vi "GEOM_AbsROI.vi"(10 "readmode":string) -> ()   [LabVIEW 2016]
uses:
  GEOM_VAR_action.ctl
  GEOM_Gbls.vi
  DBSHAND/private/vis/DatabaseHand_Element_Set(string).vi
  DBSHAND/private/vis/DatabaseHand_Element_Set(U32).vi
panel:
  out "ysize out":u32
  out "ystart out":u32
  out "xsize out":u32
  out "xstart out":u32
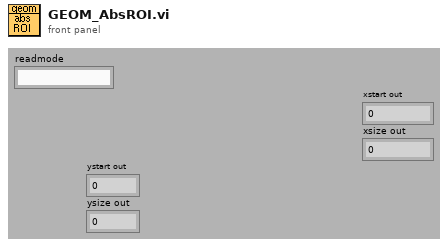
[diagram p1: front panel]
types:
  T1 = typedef "GEOM_FPAReadMode.ctl" = cluster{"name":string, "Amplifiers":T2[]}
  T2 = typedef "GEOM_Amplifier.ctl" = cluster{"number":i32, "type":T3, "rotated":i16, "fliped":u16, "FPAcoord":cluster{"xstart":i32, "ystart":i32}, "Physical_size":cluster{"columns":i32, "rows":i32}, "predata":cluster{"columns":i32, "rows":i32}, "postdata":cluster{"columns":i32, "rows":i32}, "Req ROIs":T4, "Corr ROI":T4, "Detnumber":i32, "ampID":string, "discard":i32}
  T3 = typedef "GEOM_AmpType.ctl" = u16
  T4 = typedef "GEOM_ROI.ctl" = T5[]
  T5 = typedef "GEOM_Coords.ctl" = cluster{"xstart":u32, "ystart":u32, "xsize":u32, "ysize":u32}
  T6 = typedef "GEOM_VAR_action.ctl" = enum16{"read", "write"}
  T7 = cluster{"xstart":i32, "ystart":i32, "xend":i32, "yend":i32}
  T8 = typedef "DatabaseHand_RefNum.ctl" = refnum<vi>
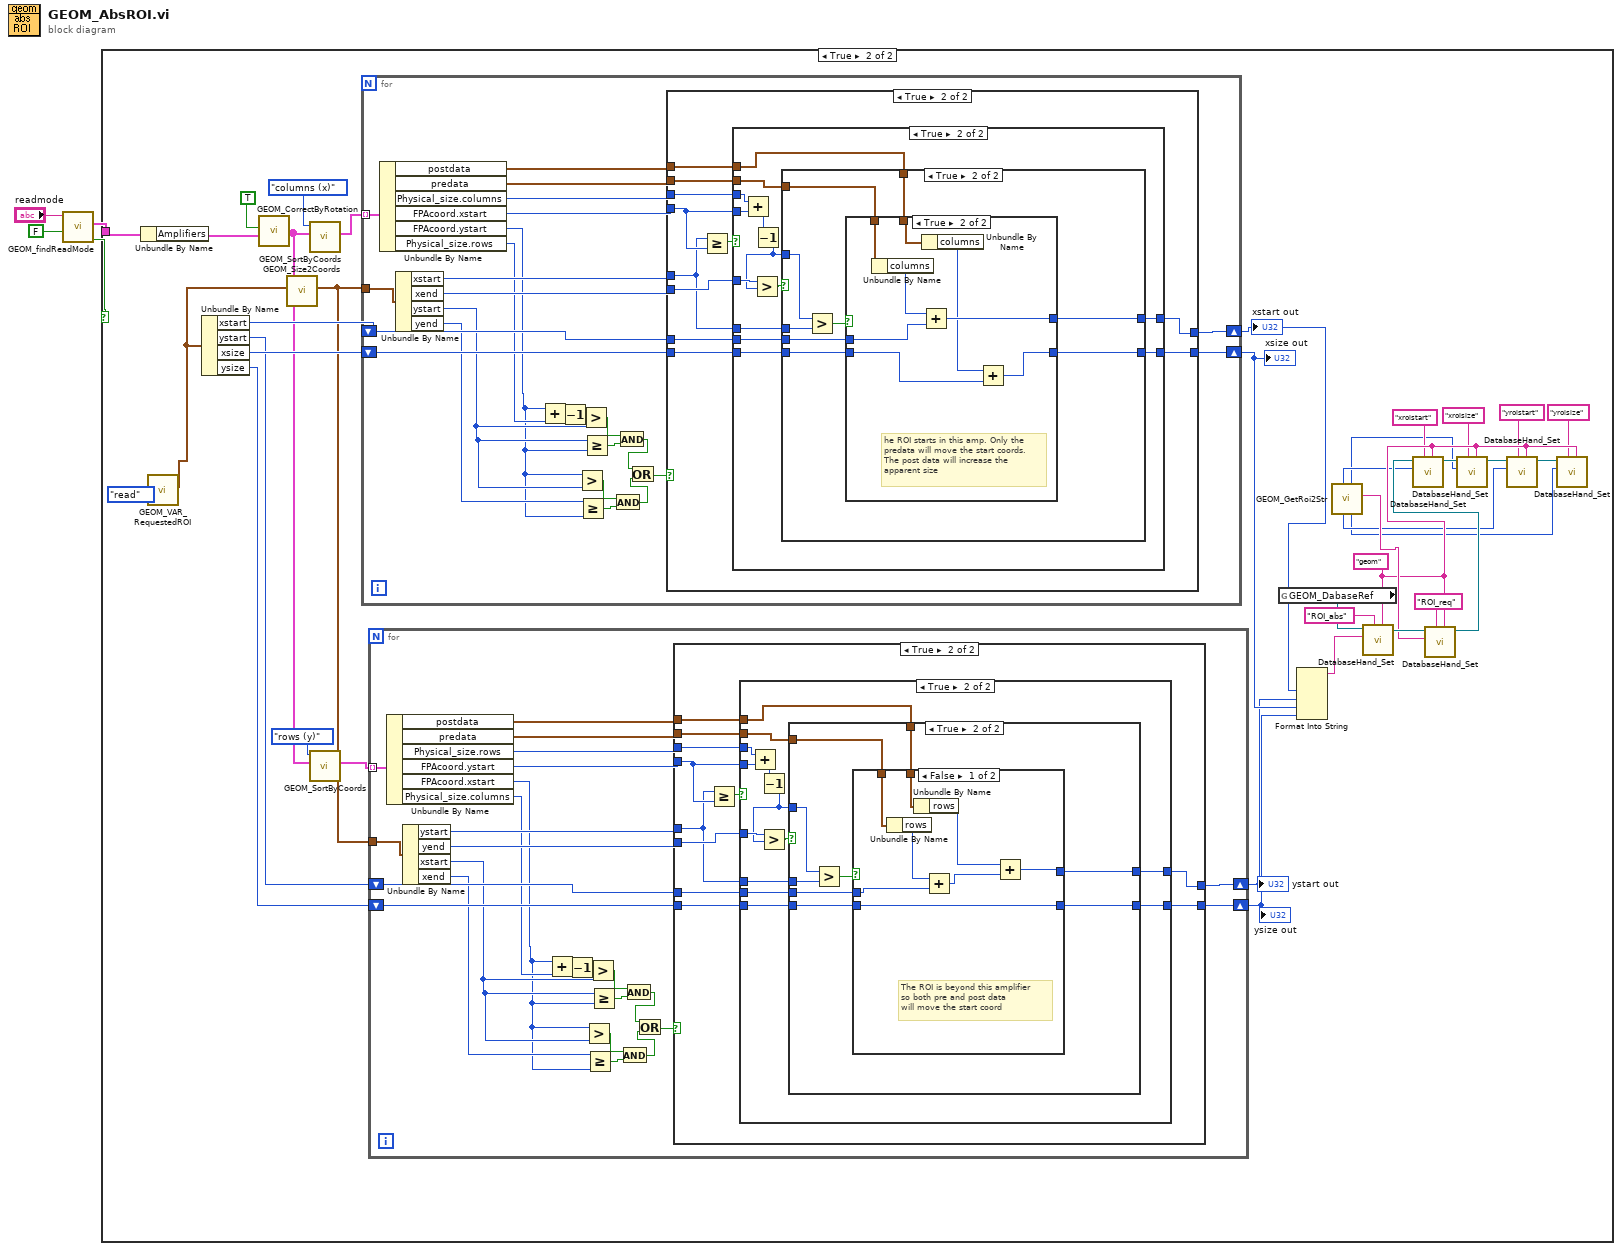
[diagram p0: block diagram]
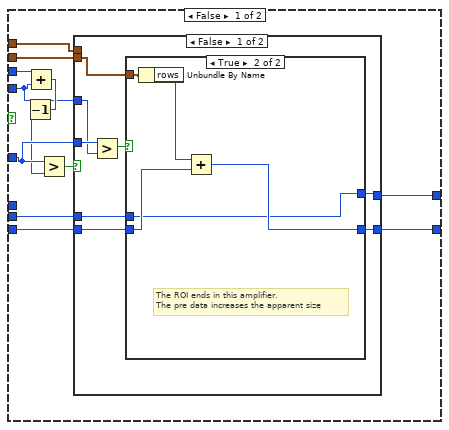
[diagram p4: hidden frame]
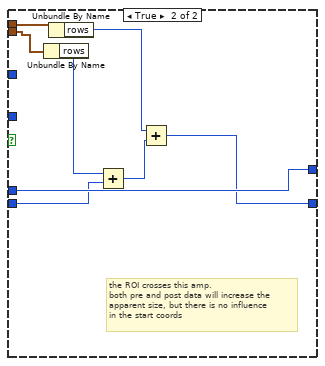
[diagram p6: hidden frame]
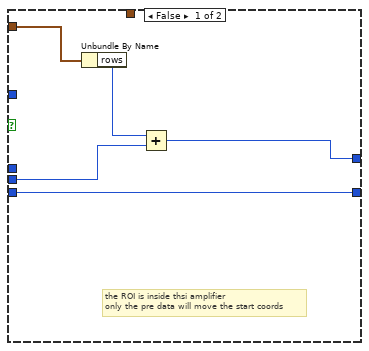
[diagram p7: hidden frame]
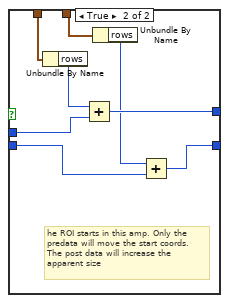
[diagram p8: hidden frame]
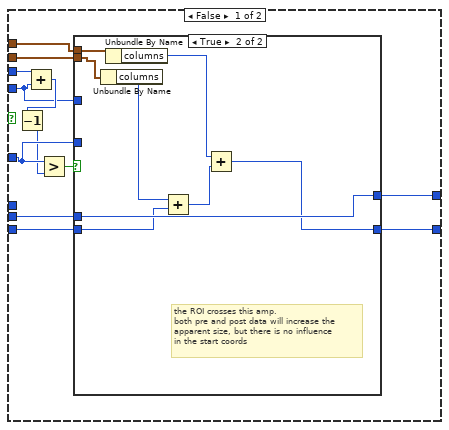
[diagram p10: hidden frame]
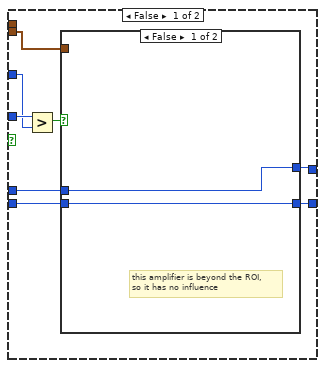
[diagram p11: hidden frame]
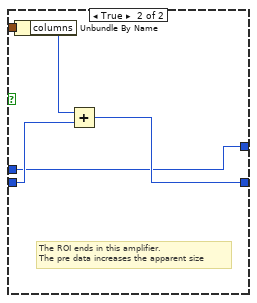
[diagram p12: hidden frame]
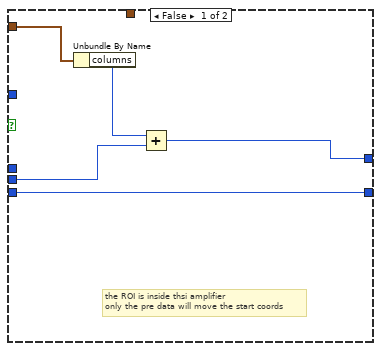
[diagram p13: hidden frame]
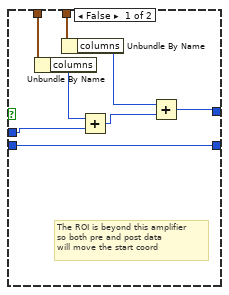
[diagram p14: hidden frame]
diagram:
  n1 = call "GEOM_findReadMode.vi"("binning corrected?"=FALSE, "readmode"="readmode") -> ("corramp found"=w2:bool, "FPAReadMode"=w1:T1)  [unwired: 1 in, 7 out]
  n2 = case shown="True" w2 {
    tunnel: w1 -> [_ w41]
    frame False {
    }
    frame True {
      w13 = "geom" ("group")
      n3 = Unbundle By Name(w41) -> ("Amplifiers"=w40:T2[])
      n4 = call "GEOM_VAR_RequestedROI.vi"("Action"=GEOM_VAR_action."read") -> ("GEOM_RequestedROI out"=w22:T5)  [unwired: 1 in, 9 out]
      n5 = Unbundle By Name(w22) -> ("xstart"=w38:u32, "ystart"=w31:u32, "xsize"=w36:u32, "ysize"=w30:u32)
      n6 = call "GEOM_CorrectByRotation.vi"("Amplifiers"=w40, "rotate ROIs?"=TRUE) -> ("rotated amps"=w35:T2[])  [unwired: 9 out]
      n7 = call "GEOM_Size2Coords.vi"("Size"=w22) -> ("Coords"=w32:T7)  [unwired: 10 out]
      n8 = call "GEOM_SortByCoords.vi"("amplifiers"=w35, "how"=enum16{"rows (y)", "columns (x)"}."columns (x)") -> ("sorted amplifiers"=w37:T2[])  [unwired: 9 out]
      n9 = call "GEOM_SortByCoords.vi"("amplifiers"=w35, "how"=enum16{"rows (y)", "columns (x)"}."rows (y)") -> ("sorted amplifiers"=w33:T2[])  [unwired: 9 out]
      n10 = for {
        shift-right: [w180] -> w27
        shift-left: w38 -> [w181]
        tunnel: w37 -> [w183] mode=indexing
        tunnel: w32 -> [w182]
        shift-right: [w172] -> w26
        shift-left: w36 -> [w173]
        n11 = Unbundle By Name(w183) -> ("postdata"=w175:cluster{"columns":i32, "rows":i32}, "predata"=w176:cluster{"columns":i32, "rows":i32}, "Physical_size.columns"=w177:i32, "FPAcoord.xstart"=w179:i32, "FPAcoord.ystart"=w160:i32, "Physical_size.rows"=w166:i32)
        n12 = Unbundle By Name(w182) -> ("xstart"=w178:i32, "xend"=w174:i32, "ystart"=w162:i32, "yend"=w161:i32)
        n13 = Add(x=w160, y=w166) -> (x+y=w171:i32)
        n14 = Decrement(x=w171) -> (x-1=w159:i32)
        n15 = Greater?(x=w160, y=w162) -> (0:w168:bool)
        n16 = Greater Or Equal?(x=w161, y=w160) -> (x >= y?=w167:bool)
        n17 = Greater?(x=w159, y=w162) -> (0:w170:bool)
        n18 = Greater Or Equal?(x=w162, y=w160) -> (x >= y?=w169:bool)
        n19 = And(x=w168, y=w167) -> (x .and. y?=w164:bool)
        n20 = And(x=w170, y=w169) -> (x .and. y?=w163:bool)
        n21 = Or(x=w163, y=w164) -> (x .or. y?=w165:bool)
        n22 = case shown="True" w165 {
          tunnel: w181 -> [w185 w190]
          tunnel: [w185 w189] -> w180
          tunnel: w179 -> [_ w194]
          tunnel: w178 -> [_ w192]
          tunnel: w177 -> [_ w193]
          tunnel: w176 -> [_ w191]
          tunnel: w175 -> [_ w188]
          tunnel: w174 -> [_ w195]
          tunnel: w173 -> [w184 w187]
          tunnel: [w184 w186] -> w172
          frame False {
            # "the ROI is above this amp, so it has no effect"
          }
          frame True {
            n23 = Greater Or Equal?(x=w192, y=w194) -> (x >= y?=w196:bool)
            n24 = case shown="True" w196 {
              tunnel: w195 -> [w199 w244]
              tunnel: w194 -> [w198 w243]
              tunnel: w193 -> [w208 w242]
              tunnel: w192 -> [_ w239]
              tunnel: w191 -> [w204 w238]
              tunnel: w190 -> [w203 w237]
              tunnel: [w202 w236] -> w189
              tunnel: w188 -> [w205 w235]
              tunnel: w187 -> [w201 w234]
              tunnel: [w200 w233] -> w186
              frame False {
                n25 = Add(x=w208, y=w198) -> (x+y=w207:i32)
                n26 = Decrement(x=w207) -> (x-1=w197:i32)
                n27 = Greater?(x=w199, y=w197) -> (0:w206:bool)
                n28 = case shown="True" w206 {
                  tunnel: w205 -> [_ w231]
                  tunnel: w204 -> [w216 w230]
                  tunnel: w203 -> [w210 w226]
                  tunnel: [w209 w226] -> w202
                  tunnel: w201 -> [w215 w225]
                  tunnel: [w214 w224] -> w200
                  tunnel: w199 -> [w213 _]
                  tunnel: w198 -> [w212 _]
                  frame False {
                    n29 = Greater?(x=w213, y=w212) -> (0:w211:bool)
                    n30 = case shown="False" w211 {
                      tunnel: w216 -> [_ w223]
                      tunnel: w215 -> [w218 w222]
                      tunnel: [w218 w220] -> w214
                      tunnel: w210 -> [w217 w219]
                      tunnel: [w217 w219] -> w209
                      frame False {
                        # "this amplifier is beyond the ROI,\nso it has no influence"
                      }
                      frame True {
                        # "The ROI ends in this amplifier.\nThe pre data increases the apparent size"
                        n31 = Unbundle By Name(w223) -> ("columns"=w221:i32)
                        n32 = Add(x=w221, y=w222) -> (x+y=w220:u32)
                      }
                    }
                  }
                  frame True {
                    # "the ROI crosses this amp.\nboth pre and post data will increase the \napparent size, but there is no influence\nin the start coords"
                    n33 = Unbundle By Name(w230) -> ("columns"=w229:i32)
                    n34 = Unbundle By Name(w231) -> ("columns"=w228:i32)
                    n35 = Add(x=w229, y=w225) -> (x+y=w227:u32)
                    n36 = Add(x=w228, y=w227) -> (x+y=w224:u32)
                  }
                }
              }
              frame True {
                n37 = Add(x=w242, y=w243) -> (x+y=w240:i32)
                n38 = Decrement(x=w240) -> (x-1=w232:i32)
                n39 = Greater?(x=w244, y=w232) -> (0:w241:bool)
                n40 = case shown="True" w241 {
                  tunnel: w232 -> [_ w258]
                  tunnel: w239 -> [_ w257]
                  tunnel: w238 -> [w249 w255]
                  tunnel: w237 -> [w248 w254]
                  tunnel: [w246 w253] -> w236
                  tunnel: w235 -> [_ w252]
                  tunnel: w234 -> [w245 w251]
                  tunnel: [w245 w250] -> w233
                  frame False {
                    # "the ROI is inside thsi amplifier\nonly the pre data will move the start coords"
                    n41 = Unbundle By Name(w249) -> ("columns"=w247:i32)
                    n42 = Add(x=w247, y=w248) -> (x+y=w246:u32)
                  }
                  frame True {
                    n43 = Greater?(x=w258, y=w257) -> (0:w256:bool)
                    n44 = case shown="True" w256 {
                      tunnel: w255 -> [w266 w274]
                      tunnel: w254 -> [w264 w272]
                      tunnel: [w260 w271] -> w253
                      tunnel: w252 -> [w265 w270]
                      tunnel: w251 -> [w259 w268]
                      tunnel: [w259 w267] -> w250
                      frame False {
                        # "The ROI is beyond this amplifier\nso both pre and post data\nwill move the start coord"
                        n45 = Unbundle By Name(w266) -> ("columns"=w263:i32)
                        n46 = Unbundle By Name(w265) -> ("columns"=w261:i32)
                        n47 = Add(x=w263, y=w264) -> (x+y=w262:u32)
                        n48 = Add(x=w261, y=w262) -> (x+y=w260:u32)
                      }
                      frame True {
                        # "he ROI starts in this amp. Only the\npredata will move the start coords.\nThe post data will increase the \napparent size"
                        n49 = Unbundle By Name(w274) -> ("columns"=w273:i32)
                        n50 = Add(x=w273, y=w272) -> (x+y=w271:u32)
                        n51 = Unbundle By Name(w270) -> ("columns"=w269:i32)
                        n52 = Add(x=w269, y=w268) -> (x+y=w267:u32)
                      }
                    }
                  }
                }
              }
            }
          }
        }
      }
      "xstart out" <- w27
      "xsize out" <- w26
      n53 = for {
        shift-right: [w64] -> w25
        shift-left: w31 -> [w65]
        tunnel: w33 -> [w67] mode=indexing
        tunnel: w32 -> [w66]
        shift-right: [w56] -> w24
        shift-left: w30 -> [w57]
        n54 = Unbundle By Name(w67) -> ("postdata"=w59:cluster{"columns":i32, "rows":i32}, "predata"=w60:cluster{"columns":i32, "rows":i32}, "Physical_size.rows"=w61:i32, "FPAcoord.ystart"=w63:i32, "FPAcoord.xstart"=w44:i32, "Physical_size.columns"=w50:i32)
        n55 = Unbundle By Name(w66) -> ("ystart"=w62:i32, "yend"=w58:i32, "xstart"=w46:i32, "xend"=w45:i32)
        n56 = Add(x=w44, y=w50) -> (x+y=w55:i32)
        n57 = Decrement(x=w55) -> (x-1=w43:i32)
        n58 = Greater?(x=w44, y=w46) -> (0:w52:bool)
        n59 = Greater Or Equal?(x=w45, y=w44) -> (x >= y?=w51:bool)
        n60 = Greater?(x=w43, y=w46) -> (0:w54:bool)
        n61 = Greater Or Equal?(x=w46, y=w44) -> (x >= y?=w53:bool)
        n62 = And(x=w52, y=w51) -> (x .and. y?=w48:bool)
        n63 = And(x=w54, y=w53) -> (x .and. y?=w47:bool)
        n64 = Or(x=w47, y=w48) -> (x .or. y?=w49:bool)
        n65 = case shown="True" w49 {
          tunnel: w65 -> [w69 w74]
          tunnel: [w69 w73] -> w64
          tunnel: w63 -> [_ w78]
          tunnel: w62 -> [_ w76]
          tunnel: w61 -> [_ w77]
          tunnel: w60 -> [_ w75]
          tunnel: w59 -> [_ w72]
          tunnel: w58 -> [_ w79]
          tunnel: w57 -> [w68 w71]
          tunnel: [w68 w70] -> w56
          frame False {
            # "the ROI is above this amp, so it has no effect"
          }
          frame True {
            n66 = Greater Or Equal?(x=w76, y=w78) -> (x >= y?=w80:bool)
            n67 = case shown="True" w80 {
              tunnel: w79 -> [w83 w128]
              tunnel: w78 -> [w82 w127]
              tunnel: w77 -> [w92 w126]
              tunnel: w76 -> [_ w123]
              tunnel: w75 -> [w88 w122]
              tunnel: w74 -> [w87 w121]
              tunnel: [w86 w120] -> w73
              tunnel: w72 -> [w89 w119]
              tunnel: w71 -> [w85 w118]
              tunnel: [w84 w117] -> w70
              frame False {
                n68 = Add(x=w92, y=w82) -> (x+y=w91:i32)
                n69 = Decrement(x=w91) -> (x-1=w81:i32)
                n70 = Greater?(x=w83, y=w81) -> (0:w90:bool)
                n71 = case shown="False" w90 {
                  tunnel: w89 -> [_ w115]
                  tunnel: w88 -> [w100 w114]
                  tunnel: w87 -> [w94 w110]
                  tunnel: [w93 w110] -> w86
                  tunnel: w85 -> [w99 w109]
                  tunnel: [w98 w108] -> w84
                  tunnel: w83 -> [w97 _]
                  tunnel: w82 -> [w96 _]
                  frame False {
                    n72 = Greater?(x=w97, y=w96) -> (0:w95:bool)
                    n73 = case shown="True" w95 {
                      tunnel: w100 -> [_ w107]
                      tunnel: w99 -> [w102 w106]
                      tunnel: [w102 w104] -> w98
                      tunnel: w94 -> [w101 w103]
                      tunnel: [w101 w103] -> w93
                      frame False {
                        # "this amplifier is beyond the ROI,\nso it has no influence"
                      }
                      frame True {
                        # "The ROI ends in this amplifier.\nThe pre data increases the apparent size"
                        n74 = Unbundle By Name(w107) -> ("rows"=w105:i32)
                        n75 = Add(x=w105, y=w106) -> (x+y=w104:u32)
                      }
                    }
                  }
                  frame True {
                    # "the ROI crosses this amp.\nboth pre and post data will increase the \napparent size, but there is no influence\nin the start coords"
                    n76 = Unbundle By Name(w114) -> ("rows"=w113:i32)
                    n77 = Unbundle By Name(w115) -> ("rows"=w112:i32)
                    n78 = Add(x=w113, y=w109) -> (x+y=w111:u32)
                    n79 = Add(x=w112, y=w111) -> (x+y=w108:u32)
                  }
                }
              }
              frame True {
                n80 = Add(x=w126, y=w127) -> (x+y=w124:i32)
                n81 = Decrement(x=w124) -> (x-1=w116:i32)
                n82 = Greater?(x=w128, y=w116) -> (0:w125:bool)
                n83 = case shown="True" w125 {
                  tunnel: w116 -> [_ w142]
                  tunnel: w123 -> [_ w141]
                  tunnel: w122 -> [w133 w139]
                  tunnel: w121 -> [w132 w138]
                  tunnel: [w130 w137] -> w120
                  tunnel: w119 -> [_ w136]
                  tunnel: w118 -> [w129 w135]
                  tunnel: [w129 w134] -> w117
                  frame False {
                    # "the ROI is inside thsi amplifier\nonly the pre data will move the start coords"
                    n84 = Unbundle By Name(w133) -> ("rows"=w131:i32)
                    n85 = Add(x=w131, y=w132) -> (x+y=w130:u32)
                  }
                  frame True {
                    n86 = Greater?(x=w142, y=w141) -> (0:w140:bool)
                    n87 = case shown="False" w140 {
                      tunnel: w139 -> [w150 w158]
                      tunnel: w138 -> [w148 w156]
                      tunnel: [w144 w155] -> w137
                      tunnel: w136 -> [w149 w154]
                      tunnel: w135 -> [w143 w152]
                      tunnel: [w143 w151] -> w134
                      frame False {
                        # "The ROI is beyond this amplifier\nso both pre and post data\nwill move the start coord"
                        n88 = Unbundle By Name(w150) -> ("rows"=w147:i32)
                        n89 = Unbundle By Name(w149) -> ("rows"=w145:i32)
                        n90 = Add(x=w147, y=w148) -> (x+y=w146:u32)
                        n91 = Add(x=w145, y=w146) -> (x+y=w144:u32)
                      }
                      frame True {
                        # "he ROI starts in this amp. Only the\npredata will move the start coords.\nThe post data will increase the \napparent size"
                        n92 = Unbundle By Name(w158) -> ("rows"=w157:i32)
                        n93 = Add(x=w157, y=w156) -> (x+y=w155:u32)
                        n94 = Unbundle By Name(w154) -> ("rows"=w153:i32)
                        n95 = Add(x=w153, y=w152) -> (x+y=w151:u32)
                      }
                    }
                  }
                }
              }
            }
          }
        }
      }
      "ystart out" <- w25
      "ysize out" <- w24
      n96 = global read "GEOM_Gbls.vi" "GEOM_DabaseRef"() -> (w29:T8)
      n97 = Format Into String(w27, w25, w26, w24) -> (resulting string=w23:string)  [unwired: 3 in, 1 out]
      n98 = call "GEOM_GetRoi2Str.vi"() -> ("roi"=w18:string, "ysize"=w5:u32, "xsize"=w7:u32, "ystart"=w6:u32, "xstart"=w8:u32)  [unwired: 7 out]
      n99 = call-poly "DatabaseHand_Set.vi"("group"=w13, "name"="ROI_abs", "value"=w23, "Database RefNum in"=w29) -> ("Database RefNum out"=w20:T8)  [unwired: 4 in, 3 out]
      n100 = call-poly "DatabaseHand_Set.vi"("group"=w13, "name"="ROI_req", "value"=w18, "Database RefNum in"=w20) -> ("Database RefNum out"=w17:T8)  [unwired: 4 in, 3 out]
      n101 = call-poly "DatabaseHand_Set.vi"("group"=w13, "name"="xroistart", "value"=w8, "Database RefNum in"=w17) -> ("Database RefNum out"=w16:T8)  [unwired: 4 in, 3 out]
      n102 = call-poly "DatabaseHand_Set.vi"("group"=w13, "name"="xroisize", "value"=w7, "Database RefNum in"=w16) -> ("Database RefNum out"=w15:T8)  [unwired: 4 in, 3 out]
      n103 = call-poly "DatabaseHand_Set.vi"("group"=w13, "name"="yroistart", "value"=w6, "Database RefNum in"=w15) -> ("Database RefNum out"=w14:T8)  [unwired: 4 in, 3 out]
      n104 = call-poly "DatabaseHand_Set.vi"("group"=w13, "name"="yroisize", "value"=w5, "Database RefNum in"=w14) -> ()  [unwired: 4 in, 4 out]
    }
  }
